vi "PROJECT_InitLogging.vi"(8 "error in":errorcluster) -> (0 "error out":errorcluster)   [LabVIEW 2022 SP3, in "Project.lvlib"]
doc: "Initiate the logging functions.\n\n____\nHAMPEL SOFTWARE ENGINEERING v2.6.0 (2023-12-19 10:54)"
uses:
  Project.lvlib
  <vilib>/Hampel Software Engineering/HSE Logger/LogLevel.ctl
  Libraries/hse-libraries/Source/hse-application/hse-application.lvclass/hse-application.ctl
  Libraries/hse-libraries/Source/hse-application/HSE Application not initialized--error.vi
  <vilib>/Utility/error.llb/Clear Errors.vi
  <vilib>/Hampel Software Engineering/HSE Logger/Handler/FileHandler/FileHandler.lvclass
  C:/Program Files/National Instruments/LabVIEW 2022/vi.lib/Hampel Software Engineering/HSE Logger/Handler/Handler.lvclass
  <vilib>/Hampel Software Engineering/HSE Logger/Handler/UserEventHandler/UserEventHandler.lvclass
  Libraries/hse-libraries/Source/hse-application/hse-application__GetSingleton.vi
  <vilib>/Utility/sysdir.llb/Get System Directory.vi
  <vilib>/Utility/error.llb/Error Cluster From Error Code.vi
  Libraries/hse-libraries/Source/hse-configuration/config-ini/config-ini.lvclass
  Libraries/hse-libraries/Source/hse-application/hse-application.lvclass
  <vilib>/Hampel Software Engineering/HSE Logger/hse-logger.lvlib
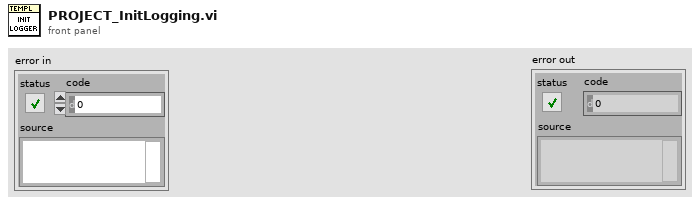
[diagram p1: front panel]
types:
  T1 = typedef "hse-logger.lvlib/LogLevel.ctl" = enum16{"DEBUG", "INFO", "WARNING", "ERROR", "CRITICAL"}
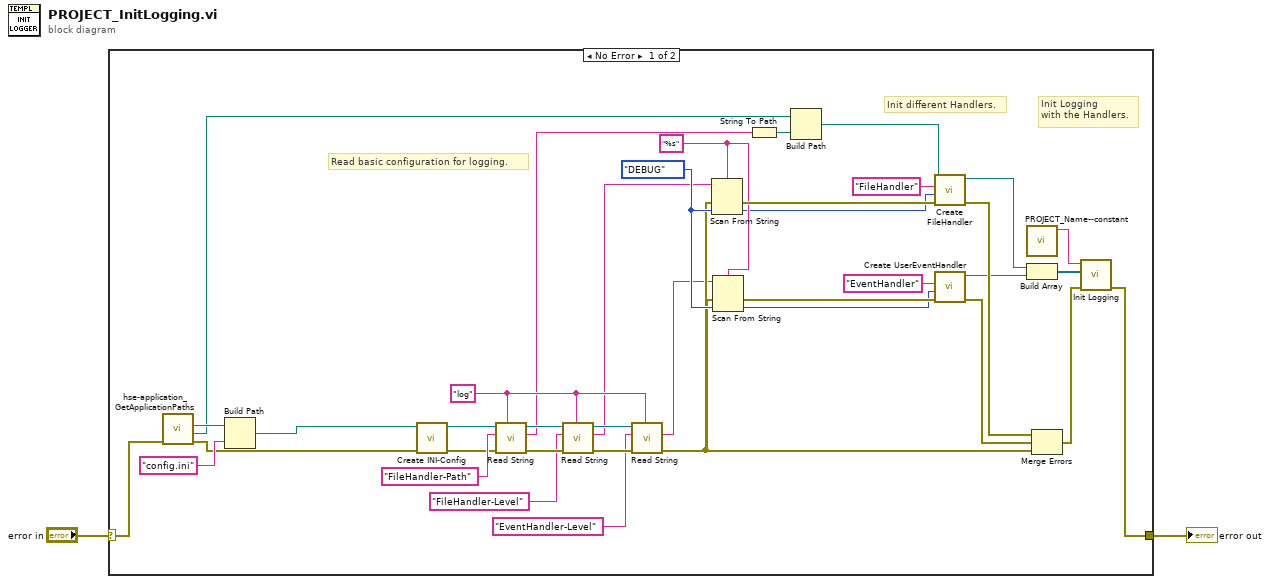
[diagram p0: block diagram]
diagram:
  n1 = case shown="No Error" "error in" {
    selector: "error in" -> [w35 w41]
    tunnel: [w16 w41] -> w1
    frame No Error {
      w25 = "%s" ("format string")
      w26 = LogLevel."DEBUG" ("Level")
      w28 = "log" ("Section")
      # "Init Logging\nwith the Handlers."
      # "Init different Handlers."
      # "Read basic configuration for logging."
      n2 = call "hse-application_GetApplicationPaths.vi"("error in"=w35) -> ("error out"=w6:errorcluster, "Data Directory"=w14:path, "Config Directory"=w36:path)  [unwired: 4 in, 4 out]
      n3 = Build Path(base path=w36, name or relative path="config.ini" ("Name")) -> (appended path=w8:path)
      n4 = call "Create INI-Config.vi"("error in"=w6, "INI Filepath"=w8) -> ("error out"=w7:errorcluster, "config-ini out"=w5:refnum<class "config-ini.lvclass">)  [unwired: 8 in]
      n5 = call-dynamic "Read String.vi"("Section"=w28, "error in"=w7, "Key"="FileHandler-Path", "config-base in"=w5) -> ("error out"=w33:errorcluster, "Value"=w12:string, "config-base out"=w32:refnum<class "config-ini.lvclass">)  [unwired: 5 in]
      n6 = call-dynamic "Read String.vi"("Section"=w28, "error in"=w33, "Key"="FileHandler-Level", "config-base in"=w32) -> ("error out"=w30:errorcluster, "Value"=w10:string, "config-base out"=w29:refnum<class "config-ini.lvclass">)  [unwired: 5 in]
      n7 = call-dynamic "Read String.vi"("Section"=w28, "error in"=w30, "Key"="EventHandler-Level", "config-base in"=w29) -> ("error out"=w18:errorcluster, "Value"=w11:string)  [unwired: 5 in, 1 out]
      n8 = Scan From String(format string=w25, input string=w10, error in=w18, default 1=w26) -> (error out=w38:errorcluster, output 1=w20:T1)  [unwired: 1 in, 2 out]
      n9 = Scan From String(format string=w25, input string=w11, error in=w18, default 1=w26) -> (error out=w37:errorcluster, output 1=w3:T1)  [unwired: 1 in, 2 out]
      n10 = String To Path(string=w12) -> (path=w9:path)
      n11 = Build Path(base path=w14, name or relative path=w9) -> (appended path=w15:path)
      n12 = call <vilib>:"Create FileHandler.vi"("error in"=w38, "Level"=w20, "Name"="FileHandler", "Filepath"=w15) -> ("error out"=w39:errorcluster, "FileHandler out"=w23:refnum<class "FileHandler.lvclass">)  [unwired: 6 in]
      n13 = call <vilib>:"Create UserEventHandler.vi"("error in"=w37, "Level"=w3, "Name"="EventHandler") -> ("error out"=w40:errorcluster, "UserEventHandler out"=w22:refnum<class "UserEventHandler.lvclass">)  [unwired: 7 in]
      n14 = call "PROJECT_Name--constant.vi"() -> ("PROJECT Name"=w13:string)  [unwired: 11 in]
      n15 = Build Array(w23, w22) -> (w21:refnum<class "Handler.lvclass">[])
      n16 = Merge Errors(w39, w40, w18) -> (w17:errorcluster)
      n17 = call <vilib>:"Init Logging.vi"("error in"=w17, "Handlers"=w21, "Name"=w13) -> ("error out"=w16:errorcluster)  [unwired: 8 in]
    }
    frame Error {
    }
  }
  "error out" <- w1
